vi "dynamicsub.vi"(9 "error in (no error)":errorcluster, 10 "Dynamic":T1) -> (1 "error out":errorcluster, 2 "generateWF ok?":i32)   [LabVIEW 2015]
uses:
  Debug 2/Test_ARTS_1.dll
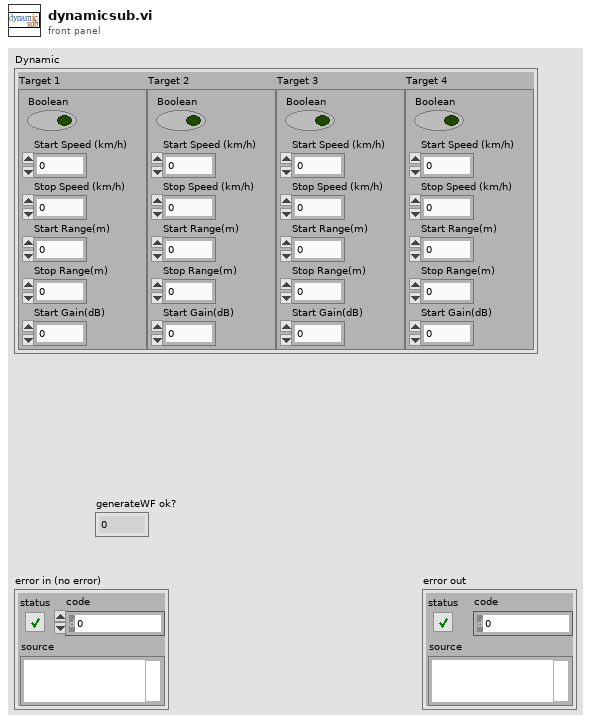
[diagram p1: front panel]
types:
  T1 = cluster{"Target 1":cluster{"Boolean":bool, "Start Speed (km/h)":dbl, "Stop Speed (km/h)":dbl, "Start Range(m)":dbl, "Stop Range(m)":dbl, "Start Gain(dB)":dbl}, "Target 2":cluster{"Boolean":bool, "Start Speed (km/h)":dbl, "Stop Speed (km/h)":dbl, "Start Range(m)":dbl, "Stop Range(m)":dbl, "Start Gain(dB)":dbl}, "Target 3":cluster{"Boolean":bool, "Start Speed (km/h)":dbl, "Stop Speed (km/h)":dbl, "Start Range(m)":dbl, "Stop Range(m)":dbl, "Start Gain(dB)":dbl}, "Target 4":cluster{"Boolean":bool, "Start Speed (km/h)":dbl, "Stop Speed (km/h)":dbl, "Start Range(m)":dbl, "Stop Range(m)":dbl, "Start Gain(dB)":dbl}}
  T2 = cluster{"Boolean":bool, "Start Speed (km/h)":dbl, "Stop Speed (km/h)":dbl, "Start Range(m)":dbl, "Stop Range(m)":dbl, "Start Gain(dB)":dbl}
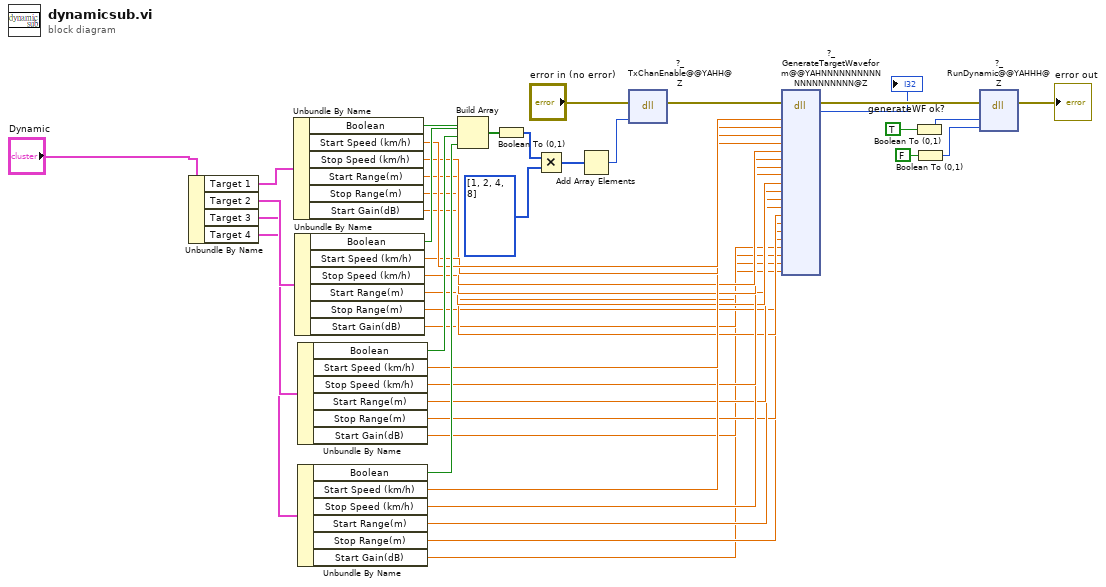
[diagram p0: block diagram]
diagram:
  n1 = Unbundle By Name("Dynamic") -> ("Target 1"=w41:T2, "Target 2"=w40:T2, "Target 3"=w39:T2, "Target 4"=w38:T2)
  n2 = Unbundle By Name(w41) -> ("Boolean"=w33:bool, "Start Speed (km/h)"=w27:dbl, "Stop Speed (km/h)"=w23:dbl, "Start Range(m)"=w19:dbl, "Stop Range(m)"=w15:dbl, "Start Gain(dB)"=w11:dbl)
  n3 = Unbundle By Name(w40) -> ("Boolean"=w32:bool, "Start Speed (km/h)"=w26:dbl, "Stop Speed (km/h)"=w22:dbl, "Start Range(m)"=w18:dbl, "Stop Range(m)"=w14:dbl, "Start Gain(dB)"=w10:dbl)
  n4 = Unbundle By Name(w39) -> ("Boolean"=w31:bool, "Start Speed (km/h)"=w25:dbl, "Stop Speed (km/h)"=w21:dbl, "Start Range(m)"=w17:dbl, "Stop Range(m)"=w13:dbl, "Start Gain(dB)"=w9:dbl)
  n5 = Unbundle By Name(w38) -> ("Boolean"=w30:bool, "Start Speed (km/h)"=w24:dbl, "Stop Speed (km/h)"=w20:dbl, "Start Range(m)"=w16:dbl, "Stop Range(m)"=w12:dbl, "Start Gain(dB)"=w8:dbl)
  n6 = Build Array(w33, w32, w31, w30) -> (w37:bool[])
  n7 = Boolean To (0,1)(Boolean=w37) -> (0, 1=w36:i16[])
  n8 = Multiply(x=w36, y=i32[] [1, 2, 4, 8]) -> (x*y=w34:i32[])
  n9 = Add Array Elements(numeric array=w34) -> (sum=w28:i32)
  n10 = dll-call lib="D:/vicomm case/cub/0717/15/Main Folder/Radar - 2015 32bit_autoqueue_angle_0319/Debug 2/Test_ARTS_1.dll" fn="?_TxChanEnable@@YAHH@Z" label="TxChanEnable"(error in="error in (no error)", "ichan"=w28) -> (error out=w29:errorcluster)  [unwired: 4 in, 1 out]
  n11 = dll-call lib="D:/vicomm case/cub/0717/15/Main Folder/Radar - 2015 32bit_autoqueue_angle_0319/Debug 2/Test_ARTS_1.dll" fn="?_GenerateTargetWaveform@@YAHNNNNNNNNNNNNNNNNNNNN@Z" label="GenerateWaveform"(error in=w29, "StartSpeedch1"=w27, "StartSpeedch2"=w26, "StartSpeedch3"=w25, "StartSpeedch4"=w24, "StopSpeedch1"=w23, "StopSpeedch2"=w22, "StopSpeedch3"=w21, "StopSpeedch4"=w20, "Startrangech1"=w19, "Startrangech2"=w18, "Startrangech3"=w17, "Startrangech4"=w16, "Stoprangech1"=w15, "Stoprangech2"=w14, "Stoprangech3"=w13, "Stoprangech4"=w12, "gaindBch1"=w11, "gaindBch2"=w10, "gaindBch3"=w9, "gaindBch4"=w8) -> (error out=w7:errorcluster, "return type"=→"generateWF ok?":i32)  [unwired: 22 in, 1 out]
  n12 = Boolean To (0,1)(Boolean=TRUE) -> (0, 1=w42:i16)
  n13 = Boolean To (0,1)(Boolean=FALSE) -> (0, 1=w43:i16)
  n14 = dll-call lib="D:/vicomm case/cub/0717/15/Main Folder/Radar - 2015 32bit_autoqueue_angle_0319/Debug 2/Test_ARTS_1.dll" fn="?_RunDynamic@@YAHHH@Z" label="RunDynamic"(error in=w7, "Cont"=w42, "exttrigger"=w43) -> (error out=→"error out":errorcluster)  [unwired: 5 in, 1 out]
